vi "merFISH_read_next_task_TDMS.vi"(3 "error in":errorcluster, 4 "Starting time":dbl, 5 "Log file":refnum<file>) -> (0 "error out":errorcluster, 2 "task":T2)   [LabVIEW 2015]
uses:
  CONTROLS/Q_main_element.ctl
  GLOBAL/Global_ABORT.vi
  GLOBAL/Global_MAIN.vi
panel:
  out "Instruction":T1(ring)
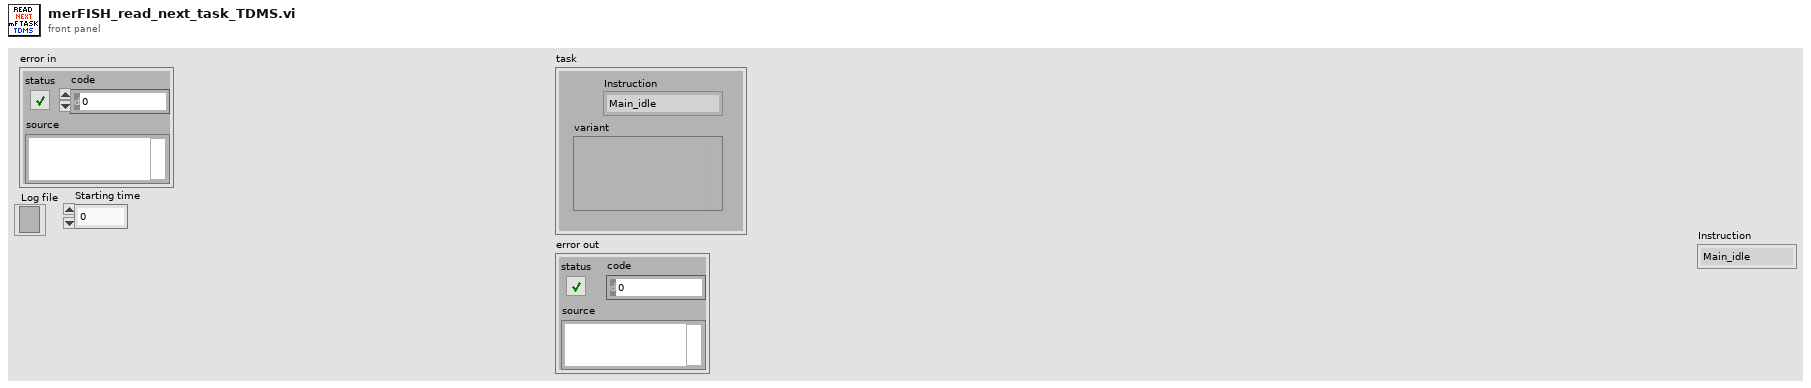
[diagram p1: front panel]
types:
  T1 = enum16{"Main_idle", "Main_initialize", "Main_initialize_TDMS", "Main_initialize_Queue", "Main_error", "Main_DAQ_initialization_results", "Main_ASI_initialization_results", "Main_Piezo_initialization_results", "Main_Valve_initialization_results", "Main_Pump_initialization_results", "Main_CAMERA_initialization_results", "Main_FPGA_initialization_results", "Main_DAQ_error", "Main_ASI_error", "Main_Piezo_error", "Main_CAMERA_error", "Main_Valve_error", "Main_Pump_error", "Main_FPGA_error", "Main_start_acquiring", "Main_not_acquiring", "Main_acquiring", "Main_stop_acquiring", "Main_change_exposure", "Main_change_z_scan_parameters", "Main_define_ROI", "Main_define_mosaic", "Main_read_kinetic_time", "Main_cooler", "Main_read_temperature", "Main_save_XY", "Main_load_XY", "Main_discard_XY", "Main_move_to_XY", "Main_measure_QPD", "Main_autofocus_calibration", "Main_autofocus_initialization", "Main_autofocus_stop", "Main_save_PID", "Main_change_H_valve_position", "Main_two_way_valve", "Main_save_movie", "Main_init_single_scan", "Main_single_scan", "Main_stop_single_scan", "Main_merFISH_illumination_parameters", "Main_merFISH_buffer_probe_list", "Main_merFISH_injections_procedure", "Main_merFISH_save_setpoint", "Main_merFISH_DAPI_parameters", "Main_merFISH_Brightfield_parameters", "Main_merFISH_save_embryo_ROI", "Main_merFISH_init", "Main_merFISH_resume", "Main_merFISH_start_autofocus", "Main_merFISH_open_close_valve_merFISH", "Main_merFISH_open_close_valve_photobleaching", "Main_merFISH_hybridization", "Main_merFISH_move_to_ROI", "Main_merFISH_wait_stabilization", "Main_merFISH_move_to_REF", "Main_merFISH_scan", "Main_merFISH_photobleaching_injection", "Main_merFISH_photobleaching", "Main_merFISH_send_email", "Main_merFISH_close", "Main_STOP"}
  T2 = typedef "Q_main_element.ctl" = cluster{"variant":variant, "Instruction":enum16{"Main_idle", "Main_initialize", "Main_initialize_TDMS", "Main_initialize_Queue", "Main_error", "Main_DAQ_initialization_results", "Main_ASI_initialization_results", "Main_Piezo_initialization_results", "Main_Valve_initialization_results", "Main_Pump_initialization_results", "Main_CAMERA_initialization_results", "Main_FPGA_initialization_results", "Main_DAQ_error", "Main_ASI_error", "Main_Piezo_error", "Main_CAMERA_error", "Main_Valve_error", "Main_Pump_error", "Main_FPGA_error", "Main_start_acquiring", "Main_not_acquiring", "Main_acquiring", "Main_stop_acquiring", "Main_change_exposure", "Main_change_z_scan_parameters", "Main_define_ROI", "Main_define_mosaic", "Main_read_kinetic_time", "Main_cooler", "Main_read_temperature", "Main_save_XY", "Main_load_XY", "Main_discard_XY", "Main_move_to_XY", "Main_measure_QPD", "Main_autofocus_calibration", "Main_autofocus_initialization", "Main_autofocus_stop", "Main_save_PID", "Main_change_H_valve_position", "Main_two_way_valve", "Main_save_movie", "Main_init_single_scan", "Main_single_scan", "Main_stop_single_scan", "Main_merFISH_illumination_parameters", "Main_merFISH_buffer_probe_list", "Main_merFISH_injections_procedure", "Main_merFISH_save_setpoint", "Main_merFISH_DAPI_parameters", "Main_merFISH_Brightfield_parameters", "Main_merFISH_save_embryo_ROI", "Main_merFISH_init", "Main_merFISH_resume", "Main_merFISH_start_autofocus", "Main_merFISH_open_close_valve_merFISH", "Main_merFISH_open_close_valve_photobleaching", "Main_merFISH_hybridization", "Main_merFISH_move_to_ROI", "Main_merFISH_wait_stabilization", "Main_merFISH_move_to_REF", "Main_merFISH_scan", "Main_merFISH_photobleaching_injection", "Main_merFISH_photobleaching", "Main_merFISH_send_email", "Main_merFISH_close", "Main_STOP"}}
  T3 = enum16{"open", "open or create", "create or replace", "create", "open (read-only)"}
  T4 = cluster{"ROI #":i32, "Probe #":i32, "Folder# ":i32, "Embryo #":i32}
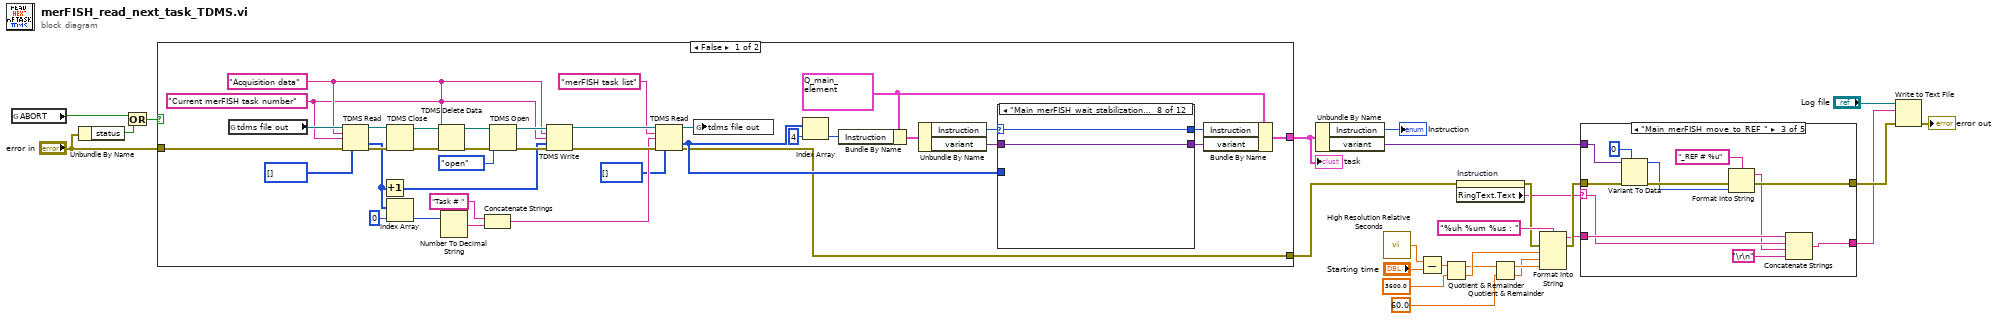
[diagram p0: block diagram]
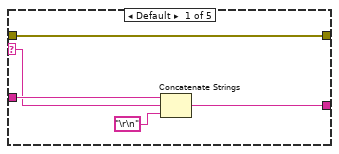
[diagram p2: hidden frame]
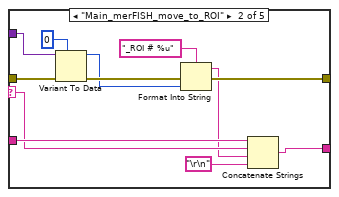
[diagram p3: hidden frame]
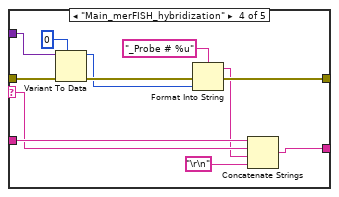
[diagram p4: hidden frame]
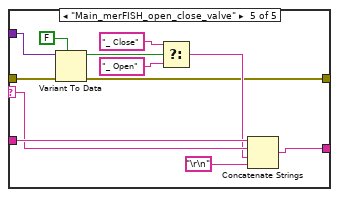
[diagram p5: hidden frame]
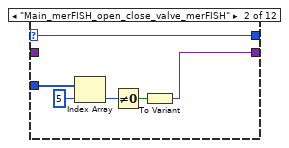
[diagram p7: hidden frame]
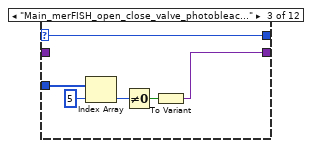
[diagram p8: hidden frame]
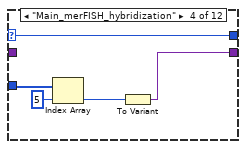
[diagram p9: hidden frame]
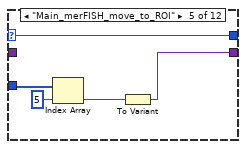
[diagram p10: hidden frame]
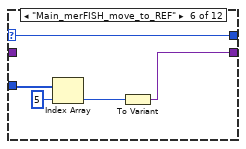
[diagram p11: hidden frame]
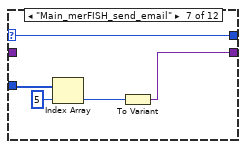
[diagram p12: hidden frame]
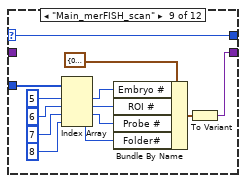
[diagram p13: hidden frame]
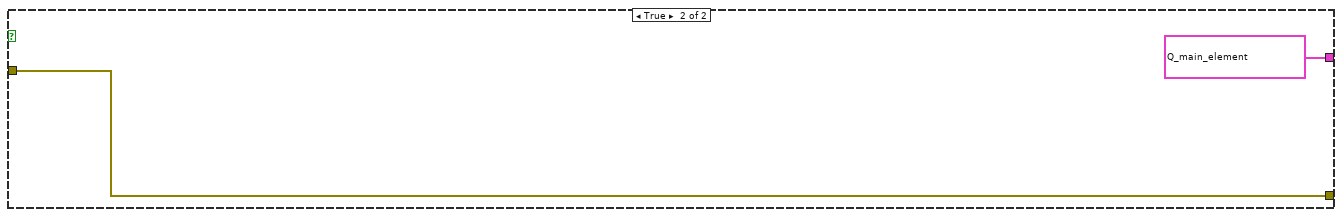
[diagram p17: hidden frame]
diagram:
  n1 = global read "Global_ABORT.vi" "ABORT"() -> (w26:bool)
  n2 = Unbundle By Name("error in") -> ("status"=w25:bool)
  n3 = Or(x=w26, y=w25) -> (x .or. y?=w23:bool)
  n4 = case shown="False" w23 {
    tunnel: "error in" -> [w30 w119]
    tunnel: [w29 T2 {"variant"=variant, "Instruction"=enum."Main_merFISH_close"} ("element")] -> w4
    tunnel: [w28 w119] -> w6
    frame False {
      w33 = T2 {"variant"=variant, "Instruction"=enum."Main_idle"} ("element")
      w52 = "Current merFISH task number" ("group name in")
      w53 = "Acquisition data" ("group name in")
      n5 = global read "Global_MAIN.vi" "tdms file out"() -> (w63:refnum<k34>)
      n6 = TDMS Read(0:w63, 5:w53, 7:w52, 11:w30, 12:u32[] [] ("appended array")) -> (4:w43:refnum<k34>, 10:w50:u32[], 15:w56:errorcluster)  [unwired: 3 in, 3 out]
      n7 = Increment(x=w50) -> (x+1=w49:u32[])
      n8 = TDMS Close(8:w56, 11:w43) -> (0:w57:errorcluster, 3:w58:path)
      n9 = Index Array(array=w50, index=0) -> (element=w46:u32)
      n10 = TDMS Delete Data(8:w57, 9:w52, 10:w53, 11:w58) -> (0:w60:errorcluster, 3:w61:path)  [unwired: 3 in]
      n11 = Number To Decimal String(number=w46) -> (decimal integer string=w47:string)  [unwired: 1 in]
      n12 = Concatenate Strings("Task # " ("string"), w47) -> (w41:string)
      n13 = TDMS Open(8:w60, 10:T3."open" ("operation (0:open)"), 11:w61) -> (0:w55:errorcluster, 3:w54:refnum<k34>)  [unwired: 4 in]
      n14 = TDMS Write(0:w54, 5:w53, 7:w52, 9:w49, 11:w55) -> (4:w45:refnum<k34>, 15:w44:errorcluster)  [unwired: 1 in, 2 out]
      n15 = TDMS Read(0:w45, 5:"merFISH task list" ("group name in (Untitled)"), 7:w41, 11:w44, 12:i32[] []) -> (4:w27:refnum<k34>, 10:w34:i32[], 15:w28:errorcluster)  [unwired: 3 in, 3 out]
      n16 = global write "Global_MAIN.vi" "tdms file out"(w27) -> ()
      n17 = Index Array(array=w34, index=4) -> (element=w38:i32)
      n18 = Bundle By Name(cluster=w33, "Instruction"=w38) -> (w37:T2)
      n19 = Unbundle By Name(w37) -> ("Instruction"=w36:T1, "variant"=w35:variant)
      n20 = case shown="\"Main_merFISH_wait_stabilization\"" w36 {
        selector: w36 -> [w65 w71 w77 w82 w87 w92 w97 w99 w112 w114 w116 w118]
        tunnel: w35 -> [w64 _ _ _ _ _ _ w98 _ w113 w115 w117]
        tunnel: [w65 w71 w77 w82 w87 w92 w97 w99 w112 w114 w116 w118] -> w32
        tunnel: [w64 w66 w72 w79 w84 w89 w94 w98 w100 w113 w115 w117] -> w31
        tunnel: w34 -> [_ w67 w73 w80 w85 w90 w95 _ w101 _ _ _]
        frame "Main_merFISH_start_autofocus" {
        }
        frame "Main_merFISH_open_close_valve_merFISH" {
          n21 = Index Array(array=w67, index=5) -> (element=w69:i32)
          n22 = Not Equal To 0?(x=w69) -> (x != 0?=w68:bool)
          n23 = To Variant(anything=w68) -> (Variant=w66:variant)
        }
        frame "Main_merFISH_open_close_valve_photobleaching" {
          n24 = Index Array(array=w73, index=5) -> (element=w75:i32)
          n25 = Not Equal To 0?(x=w75) -> (x != 0?=w74:bool)
          n26 = To Variant(anything=w74) -> (Variant=w72:variant)
        }
        frame "Main_merFISH_hybridization" {
          n27 = Index Array(array=w80, index=5) -> (element=w78:i32)
          n28 = To Variant(anything=w78) -> (Variant=w79:variant)
        }
        frame "Main_merFISH_move_to_ROI" {
          n29 = Index Array(array=w85, index=5) -> (element=w83:i32)
          n30 = To Variant(anything=w83) -> (Variant=w84:variant)
        }
        frame "Main_merFISH_move_to_REF" {
          n31 = Index Array(array=w90, index=5) -> (element=w88:i32)
          n32 = To Variant(anything=w88) -> (Variant=w89:variant)
        }
        frame "Main_merFISH_send_email" {
          n33 = Index Array(array=w95, index=5) -> (element=w93:i32)
          n34 = To Variant(anything=w93) -> (Variant=w94:variant)
        }
        frame "Main_merFISH_wait_stabilization" {
        }
        frame "Main_merFISH_scan" {
          n35 = Index Array(array=w101, index #1=5 ("index"), index #2=6 ("index"), index #3=7 ("index"), index #4=8 ("index")) -> (element #1=w108:i32, element #2=w107:i32, element #3=w106:i32, element #4=w102:i32)
          n36 = Bundle By Name(cluster=T4 {"ROI #"=0, "Probe #"=0, "Folder# "=0, "Embryo #"=0}, "Embryo #"=w108, "ROI #"=w107, "Probe #"=w106, "Folder#"=w102) -> (w105:T4)
          n37 = To Variant(anything=w105) -> (Variant=w100:variant)
        }
        frame "Main_merFISH_photobleaching_injection" {
        }
        frame "Main_merFISH_photobleaching" {
        }
        frame "Main_merFISH_close", Default {
        }
      }
      n38 = Bundle By Name(cluster=w33, "Instruction"=w32, "variant"=w31) -> (w29:T2)
    }
    frame True {
    }
  }
  "task" <- w4
  n39 = Unbundle By Name(w4) -> ("Instruction"=→"Instruction":T1, "variant"=w9:variant)
  n40 = call <vilib>:"High Resolution Relative Seconds.vi"() -> ("relative seconds"=w11:dbl)
  n41 = Subtract(x=w11, y="Starting time") -> (x-y=w12:dbl)
  n42 = Quotient & Remainder(x=w12, y=3600.0) -> (x-y*floor(x/y)=w14:dbl, floor(x/y)=w19:dbl)
  n43 = property on="Instruction" class="Enum (strict)"(error in=w6) -> (error out=w17:errorcluster, "RingText.Text"=w8:string)  [unwired: 1 in, 1 out]
  n44 = Quotient & Remainder(x=w14, y=60.0) -> (x-y*floor(x/y)=w21:dbl, floor(x/y)=w20:dbl)
  n45 = Format Into String(format string="%uh %um %us : " ("initial string"), error in=w17, w19, w20, w21) -> (resulting string=w16:string, error out=w18:errorcluster)  [unwired: 1 in]
  n46 = case shown="\"Main_merFISH_move_to_REF \"" w8 {
    selector: w8 -> [w123 w133 w145 w157 w170]
    tunnel: w16 -> [w124 w134 w146 w158 w171]
    tunnel: [w122 w127 w139 w151 w168] -> w7
    tunnel: w9 -> [_ w135 w147 w159 w172]
    tunnel: w18 -> [w121 w136 w148 w160 w173]
    tunnel: [w121 w130 w142 w154 w162] -> w10
    frame Default {
      n47 = Concatenate Strings(w124, w123, "\r\n") -> (w122:string)
    }
    frame "Main_merFISH_move_to_ROI" {
      n48 = Variant To Data(error in=w136, type=0 ("x+1"), Variant=w135) -> (data=w131:i32, error out=w132:errorcluster)
      n49 = Format Into String(format string="_ROI # %u" ("string"), error in=w132, w131) -> (resulting string=w129:string, error out=w130:errorcluster)  [unwired: 1 in]
      n50 = Concatenate Strings(w134, w133, w129, "\r\n") -> (w127:string)
    }
    frame "Main_merFISH_move_to_REF " {
      n51 = Variant To Data(error in=w148, type=0 ("x+1"), Variant=w147) -> (data=w143:i32, error out=w144:errorcluster)
      n52 = Format Into String(format string="_REF # %u" ("string"), error in=w144, w143) -> (resulting string=w141:string, error out=w142:errorcluster)  [unwired: 1 in]
      n53 = Concatenate Strings(w146, w145, w141, "\r\n") -> (w139:string)
    }
    frame "Main_merFISH_hybridization" {
      n54 = Variant To Data(error in=w160, type=0 ("x+1"), Variant=w159) -> (data=w155:i32, error out=w156:errorcluster)
      n55 = Format Into String(format string="_Probe # %u" ("string"), error in=w156, w155) -> (resulting string=w153:string, error out=w154:errorcluster)  [unwired: 1 in]
      n56 = Concatenate Strings(w158, w157, w153, "\r\n") -> (w151:string)
    }
    frame "Main_merFISH_open_close_valve" {
      n57 = Variant To Data(error in=w173, type=FALSE, Variant=w172) -> (data=w163:bool, error out=w162:errorcluster)
      n58 = Select(t="_ Close", s=w163, f="_ Open") -> (s? t:f=w164:string)
      n59 = Concatenate Strings(w171, w170, w164, "\r\n") -> (w168:string)
    }
  }
  n60 = Write to Text File(file (use dialog)="Log file", text=w7, error in=w10) -> (error out=→"error out":errorcluster)  [unwired: 1 in, 2 out]
